vi "GetType.vi"(8 "error in (no error)":errorcluster, 11 "Reset Alarms Msg":refnum<class "Reset Alarms Msg.lvclass">) -> (0 "error out":errorcluster, 2 "Data Sample":variant, 3 "Reset Alarms Msg":refnum<class "Reset Alarms Msg.lvclass">)   [LabVIEW 2016, in "LS218.lvlib" / "Reset Alarms Msg.lvclass"]
uses:
  Reset Alarms Msg.lvclass
  Reset Alarms Msg.lvclass/Reset Alarms Msg.ctl
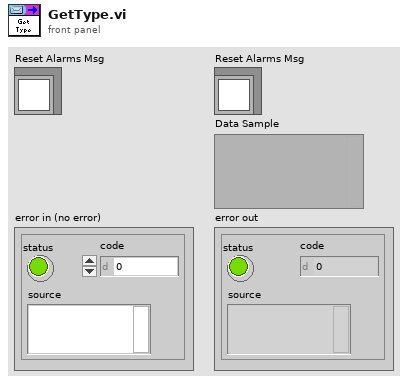
[diagram p1: front panel]
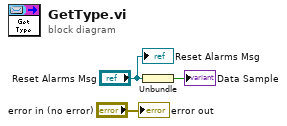
[diagram p0: block diagram]
diagram:
  n1 = Unbundle("Reset Alarms Msg") -> (→"Data Sample":bool)
  "error out" <- "error in (no error)"
  "Reset Alarms Msg" <- "Reset Alarms Msg"
